vi "Reserve Handle.vi"(6 "deadline":T1={"mode"=enum."Relative", "deadline (ms)"=30000}, 8 "error in":errorcluster, 11 "session in":refnum<class "Session.lvclass">) -> (0 "error out":errorcluster, 2 "reserved?":bool, 3 "session out":refnum<class "Session.lvclass">)   [LabVIEW 2020, in "NI_SFTP.lvlib" / "Session.lvclass"]
uses:
  <vilib>/net/SFTP/Session/Session.lvclass
  <vilib>/Utility/Deadline/Deadline.ctl
  <vilib>/Utility/Deadline/Mode.ctl
  <vilib>/net/SFTP/Session/Session.lvclass/Session.ctl
  <vilib>/Utility/Deadline/NI_Deadline.lvlib
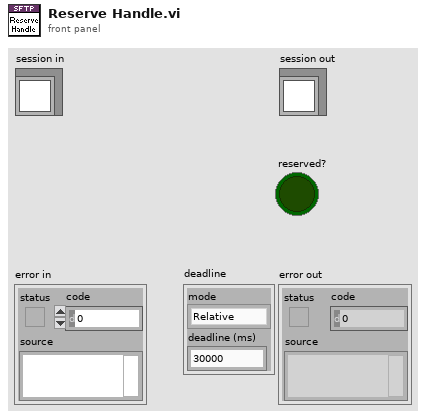
[diagram p1: front panel]
types:
  T1 = typedef "NI_Deadline.lvlib/Deadline.ctl" = cluster{"mode":T2, "deadline (ms)":u32}
  T2 = typedef "NI_Deadline.lvlib/Mode.ctl" = enum16{"Relative", "Use deadline", "Wait forever", "Nonblocking", "N/A"}
  T3 = typedef "Semaphore RefNum" = refnum<k1>
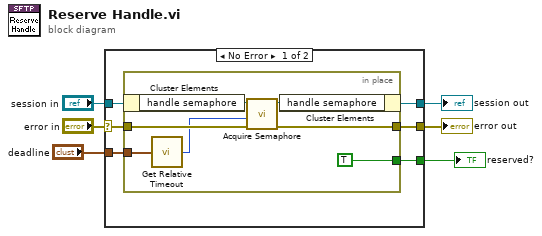
[diagram p0: block diagram]
diagram:
  n1 = case shown="No Error" "error in" {
    selector: "error in" -> [w12 w21]
    tunnel: [w11 w21] -> w5
    tunnel: [w10 w20] -> w3
    tunnel: "session in" -> [w9 w20]
    tunnel: [w8 _] -> w2
    tunnel: "deadline" -> [w7 _]
    frame No Error {
      n2 = in-place {
        in-place-border: w12 -> [w17]
        in-place-border: [w16] -> w11
        in-place-border: [TRUE ("reserved?")] -> w8
        in-place-border: w7 -> [w14]
        n3 = in-place-cluster #1(w9) -> ("handle semaphore"=w19:T3)
        n4 = call <vilib>:"Get Relative Timeout.vi"("Timeout"=w14) -> ("timeout (ms) out"=w13:i32)
        n5 = call <vilib>:"Acquire Semaphore.vi"("error in (no error)"=w17, "ms timeout (-1)"=w13, "semaphore"=w19) -> ("error out"=w16:errorcluster, "semaphore out"=w18:T3)  [unwired: 2 in, 1 out]
        n6 = in-place-cluster #1("handle semaphore"=w18) -> (w10:refnum<class "Session.lvclass">)
      }
    }
    frame Error {
    }
  }
  "error out" <- w5
  "session out" <- w3
  "reserved?" <- w2
